vi "BoolEdgeTrig.vi"(10 "Input":bool) -> (2 "Output":bool)   [LabVIEW 2016]
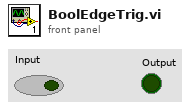
[diagram p1: front panel]
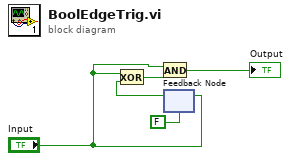
[diagram p0: block diagram]
diagram:
  n1 = feedback #1(FALSE) -> (w3:bool)
  n2 = Exclusive Or(1:w3, 2:"Input") -> (0:w5:bool)
  n3 = And(x="Input", y=w5) -> (x .and. y?=→"Output":bool)
  n4 = feedback-in #1("Input") -> ()
